vi "Add Tree Priv.vi"(0 "Tree Dictionary In":variant, 5 "Unique ID":string, 7 "Parent ID":string, 11 "Error In":errorcluster) -> (4 "Tree Dictionary Out":variant, 15 "Error Out":errorcluster)   [LabVIEW 2020, in "NI_VIAnCFGDataStructure.lvlib" / "Tree.lvclass"]
uses:
  <vilib>/addons/analyzer/VIAnCFGDataStructure/Tree Manager/Tree.lvclass
  <vilib>/addons/analyzer/VIAnCFGDataStructure/Tree Manager/Typedefs/Tree Cluster.ctl
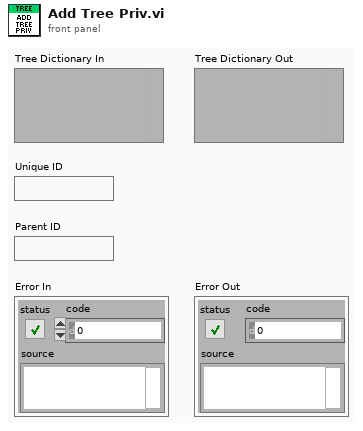
[diagram p1: front panel]
types:
  T1 = typedef "NI_VIAnCFGDataStructure.lvlib/Tree.lvclass/Tree Cluster.ctl" = cluster{"Unique ID":string, "Parent ID":string, "Child IDs":string[], "Name":string, "MetaData":string, "Data IDs":string[]}
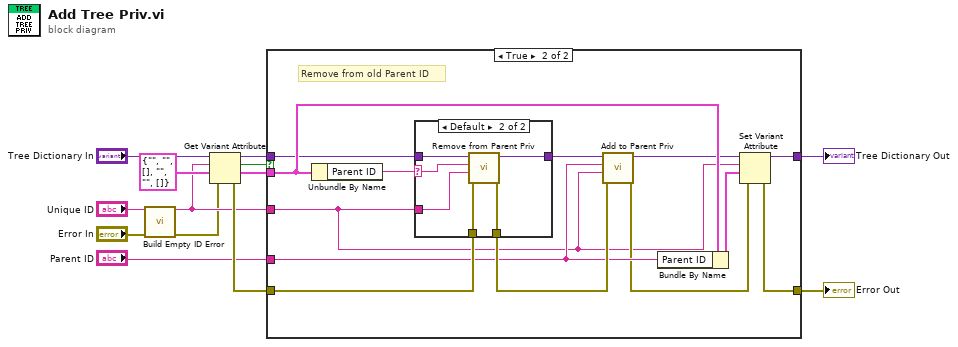
[diagram p0: block diagram]
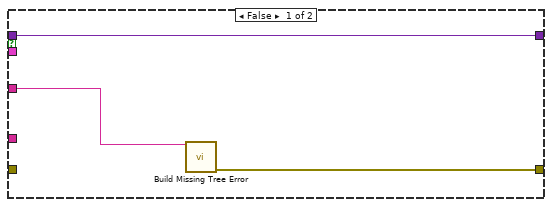
[diagram p2: hidden frame]
diagram:
  n1 = call <vilib>:"Build Empty ID Error.vi"("Unique ID"="Unique ID", "Error In"="Error In") -> ("Unique ID Out"=w2:string, "Error Out"=w1:errorcluster)  [unwired: 12 in]
  n2 = Get Variant Attribute(Variant="Tree Dictionary In", name=w2, default value (empty Variant)=T1 {"Unique ID"="", "Parent ID"="", "Child IDs"=[], "Name"="", "MetaData"="", "Data IDs"=[]} ("Cluster of class private data"), error in=w1) -> (duplicate Variant=w10:variant, found=w8:bool, value=w9:T1, error out=w11:errorcluster)
  n3 = case shown="True" w8 {
    tunnel: w9 -> [_ w27]
    tunnel: w10 -> [w16 w25]
    tunnel: w11 -> [_ w29]
    tunnel: [w14 w19] -> w12
    tunnel: [w16 w28] -> w13
    tunnel: w2 -> [w15 w18]
    tunnel: "Parent ID" -> [_ w22]
    frame False {
      n4 = call <vilib>:"Build Missing Tree Error.vi"("Unique ID"=w15) -> ("Error Out"=w14:errorcluster)  [unwired: 14 in]
    }
    frame True {
      # "Remove from old Parent ID"
      n5 = Unbundle By Name(w27) -> ("Parent ID"=w17:string)
      n6 = case shown="Default" w17 {
        selector: w17 -> [_ w32]
        tunnel: w29 -> [w30 w37]
        tunnel: w25 -> [w31 w36]
        tunnel: [w31 w35] -> w24
        tunnel: [w30 w34] -> w23
        tunnel: w18 -> [_ w33]
        frame "" {
        }
        frame Default {
          n7 = call <vilib>:"Remove from Parent Priv.vi"("Error In"=w37, "Unique ID"=w33, "Parent ID"=w32, "Tree Dictionary"=w36) -> ("Error Out"=w34:errorcluster, "Tree Dictionary Out"=w35:variant)  [unwired: 6 in]
        }
      }
      n8 = call <vilib>:"Add to Parent Priv.vi"("Error In"=w23, "Unique ID"=w18, "Parent ID"=w22, "Tree Dictionary"=w24) -> ("Error Out"=w20:errorcluster, "Tree Dictionary Out"=w21:variant)  [unwired: 6 in]
      n9 = Bundle By Name(cluster=w27, "Parent ID"=w22) -> (w26:T1)
      n10 = Set Variant Attribute(Variant=w21, name=w18, value=w26, error in=w20) -> (Variant out=w28:variant, error out=w19:errorcluster)  [unwired: 1 out]
    }
  }
  "Tree Dictionary Out" <- w13
  "Error Out" <- w12
